vi "Send Single Message To Specific Target.vi"(6 "Paras In":variant, 7 "Priority":i32, 8 "error in (no error)":errorcluster, 9 "Mail Strategy In":refnum<class "Mail Strategy.lvclass">, 10 "Message In":refnum<class "Message.lvclass">, 11 "Map Tree Queue Messenger in":refnum<class "Map Tree Queue Messenger.lvclass">) -> (0 "error out":errorcluster, 3 "Map Tree Queue Messenger out":refnum<class "Map Tree Queue Messenger.lvclass">)   [LabVIEW 2024, in "Map Tree Queue Messenger.lvclass"]
uses:
  Map Tree Queue Messenger.lvclass
  Ancestor Class/Message/Message.lvclass
  Ancestor Class/Messenger/Mail Strategy/Mail Strategy.lvclass
  Ancestor Class/Messenger/Messenger Map Composite/Messenger Map Composite.lvclass/Messenger Map Composite.ctl
  Mailman/Simple Tree Queue Mailman/Simple Tree Queue Mailman.lvclass
  Mailman/Simple Tree Queue Mailman/Simple Tree Queue Mailman.lvclass/Simple Tree Queue Mailman.ctl
  Map Tree Queue Messenger.lvclass/Map Tree Queue Messenger.ctl
  Mailman/Simple Tree Queue Mailman/Public Data/Write Address Recursive Access.vi
  Ancestor Class/Messenger/Messenger Map Composite/Public Data/Read Child Nodes.vi
  Ancestor Class/Messenger/Messenger/Messenger.lvclass
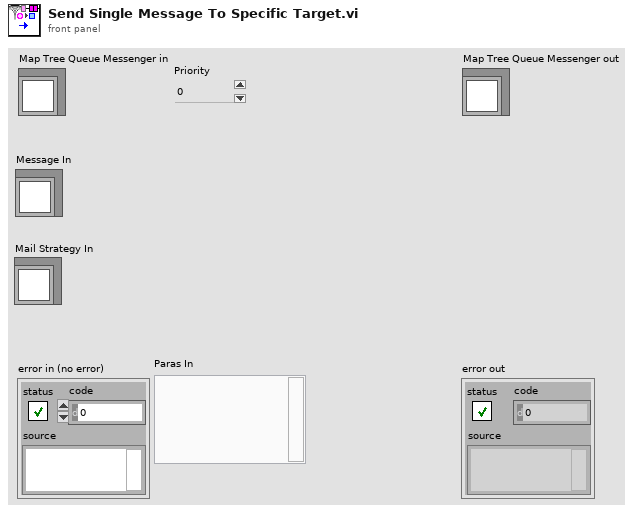
[diagram p1: front panel]
types:
  T1 = typedef "Message Queue.ctl" = refnum<queue>
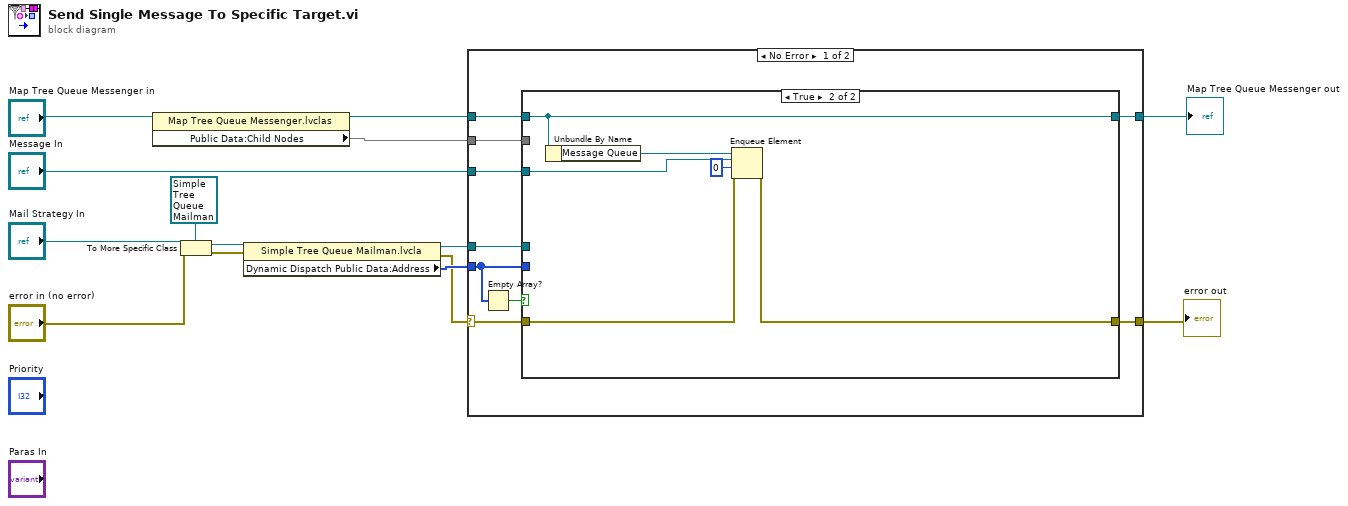
[diagram p0: block diagram]
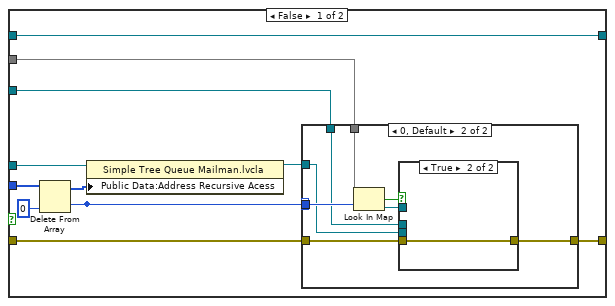
[diagram p2: hidden frame]
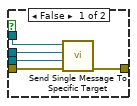
[diagram p4: hidden frame]
diagram:
  n1 = property class="Map Tree Queue Messenger.lvclas"(reference="Map Tree Queue Messenger in") -> (reference out=w9:refnum<class "Map Tree Queue Messenger.lvclass">, "Public Data:Child Nodes"=w8:map{i64, refnum<class "Messenger.lvclass">})  [unwired: 1 in, 1 out]
  n2 = To More Specific Class(target class=refnum<class "Simple Tree Queue Mailman.lvclass"> refnum ("Array Location Mailman.lvclass"), reference="Mail Strategy In", error in="error in (no error)") -> (specific class reference=w12:refnum<class "Simple Tree Queue Mailman.lvclass">, error out=w13:errorcluster)
  n3 = property class="Simple Tree Queue Mailman.lvcla"(reference=w12, error in=w13) -> (reference out=w7:refnum<class "Simple Tree Queue Mailman.lvclass">, error out=w10:errorcluster, "Dynamic Dispatch Public Data:Address"=w11:i32[])
  n4 = case shown="No Error" w10 {
    selector: w10 -> [w18 w56]
    tunnel: w9 -> [w22 w57]
    tunnel: [w20 w57] -> w6
    tunnel: [w17 w56] -> w4
    tunnel: w11 -> [w19 _]
    tunnel: "Message In" -> [w21 _]
    tunnel: w8 -> [w16 _]
    tunnel: w7 -> [w15 _]
    frame No Error {
      n5 = Empty Array?(array=w19) -> (empty?=w23:bool)
      n6 = case shown="True" w23 {
        tunnel: w22 -> [w34 w55]
        tunnel: w21 -> [w29 w53]
        tunnel: [w34 w55] -> w20
        tunnel: w19 -> [w33 _]
        tunnel: w18 -> [w31 w52]
        tunnel: [w30 w51] -> w17
        tunnel: w16 -> [w28 _]
        tunnel: w15 -> [w27 _]
        frame False {
          n7 = Delete From Array(array=w33, index=0) -> (deleted portion=w24:i32, array with subset deleted=w26:i32[])  [unwired: 1 in]
          n8 = property class="Simple Tree Queue Mailman.lvcla"(reference=w27, "Public Data:Address Recursive Acess"=w26) -> (reference out=w25:refnum<class "Simple Tree Queue Mailman.lvclass">)  [unwired: 1 in, 1 out]
          n9 = case shown="0, Default" w24 {
            tunnel: w24 -> [_ w42]
            tunnel: w31 -> [w35 w38]
            tunnel: [w35 w37] -> w30
            tunnel: w29 -> [_ w40]
            tunnel: w28 -> [_ w43]
            tunnel: w25 -> [_ w39]
            frame -2147483648..-1 {
            }
            frame 0, Default {
              n10 = Look In Map(map=w43, key=w42) -> (key not found?=w36:bool, value=w41:refnum<class "Messenger.lvclass">)  [unwired: 1 in]
              n11 = case shown="True" w36 {
                tunnel: w41 -> [w48 _]
                tunnel: w40 -> [w47 _]
                tunnel: w39 -> [w46 _]
                tunnel: w38 -> [w45 w49]
                tunnel: [w44 w49] -> w37
                frame False {
                  n12 = call-dynamic "Send Single Message To Specific Target.vi"("error in (no error)"=w45, "Mail Strategy In"=w46, "Message In"=w47, "Messenger in"=w48) -> ("error out"=w44:errorcluster)  [unwired: 6 in, 1 out]
                }
                frame True {
                }
              }
            }
          }
        }
        frame True {
          n13 = Unbundle By Name(w55) -> ("Message Queue"=w54:T1)
          n14 = Enqueue Element(queue=w54, element=w53, timeout in ms (-1)=0, error in (no error)=w52) -> (error out=w51:errorcluster)  [unwired: 2 out]
        }
      }
    }
    frame Error {
    }
  }
  "error out" <- w4
  "Map Tree Queue Messenger out" <- w6
